vi "SaveTCInfo.vi"() -> ()   [LabVIEW 2019, in "TestSeqClass.lvclass"]
uses:
  testSeq/TestSeqClass.lvclass
  testSeq/TypeDef/TestStepInfo.ctl
  TypeDef/TestInfo.ctl
panel:
  in  "error in (no error) 2":errorcluster
  in  "Save":bool
  in  "AllTestInfoSpec":T1[](array[typedef])
  in  "error in (no error)":errorcluster
  out "error out":errorcluster
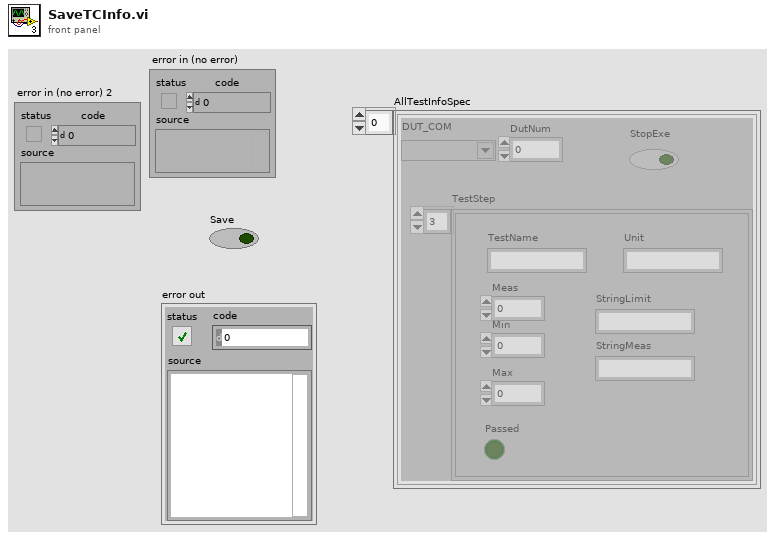
[diagram p1: front panel]
types:
  T1 = typedef "TestInfo.ctl" = cluster{"DUT_COM":refnum<visa-resource-name>, "DutNum":u16, "TestStep":T2[], "StopExe":bool}
  T2 = typedef "TestStepInfo.ctl" = cluster{"TestName":string, "Meas":dbl, "Min ":dbl, "Max":dbl, "Passed":bool, "StringLimit":string, "StringMeas":string, "Unit":string}
  T3 = enum16{"open", "open or create", "create or replace", "create", "open (read only)"}
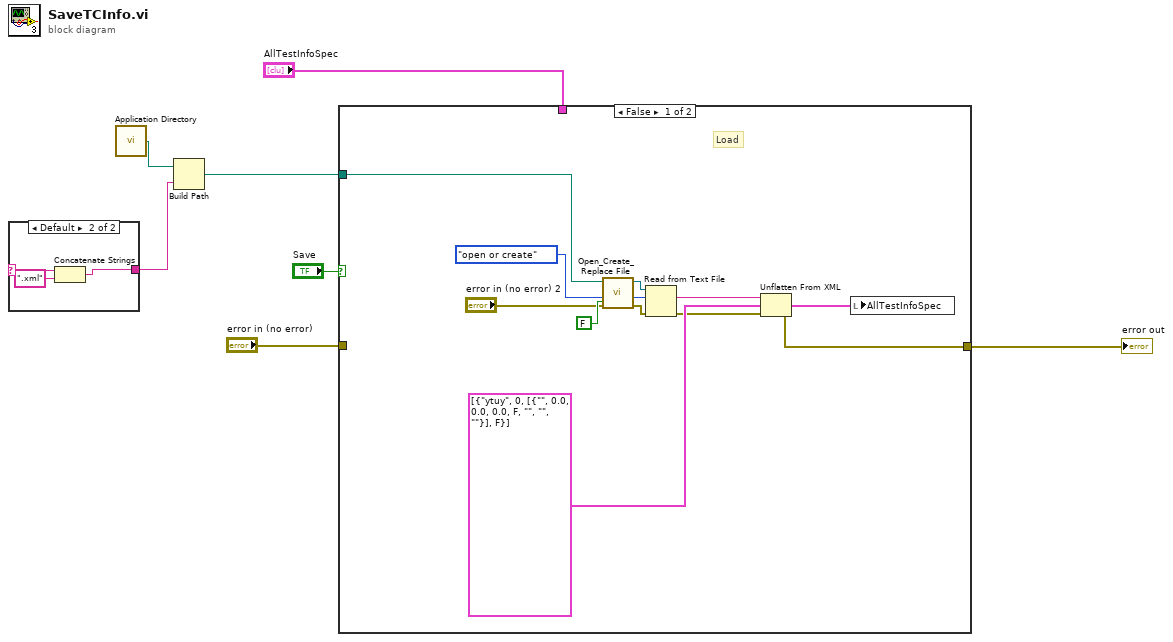
[diagram p0: block diagram]
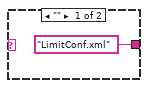
[diagram p2: hidden frame]
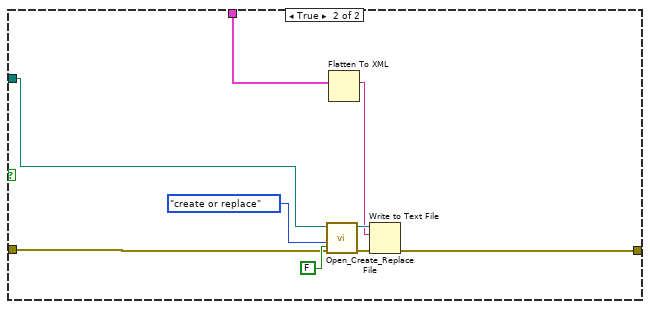
[diagram p3: hidden frame]
diagram:
  n1 = case shown="Default" {
    selector: _ -> [_ w11]
    tunnel: ["LimitConf.xml" ("name or relative path") w9] -> w1
    frame "" {
    }
    frame Default {
      n2 = Concatenate Strings(w11, ".xml" ("string")) -> (w9:string)
    }
  }
  n3 = call <vilib>:"Application Directory.vi"() -> ("Application Directory"=w2:path)
  n4 = Build Path(base path=w2, name or relative path=w1) -> (appended path=w3:path)
  n5 = case shown="False" "Save" {
    tunnel: [w13 w32] -> w7
    tunnel: "error in (no error)" -> [_ w27]
    tunnel: "AllTestInfoSpec" -> [_ w24]
    tunnel: w3 -> [w17 w26]
    frame False {
      # "Load"
      n6 = call <vilib>:"Open_Create_Replace File.vi"("advisory dialog? (display:T)"=FALSE, "error in (no error)"="error in (no error) 2", "function (open:0)"=T3."open or create", "file path"=w17) -> ("error out"=w20:errorcluster, "file size (bytes)"=w18:i32, "refnum"=w19:refnum<file>)  [unwired: 3 in, 2 out]
      n7 = Read from Text File(file (use dialog)=w19, count=w18, error in=w20) -> (text=w16:string, error out=w14:errorcluster)  [unwired: 1 in, 2 out]
      n8 = Unflatten From XML(xml string=w16, type=T1[] [{"DUT_COM"="ytuy", "DutNum"=0, "TestStep"=[{"TestName"="", "Meas"=0.0, "Min "=0.0, "Max"=0.0, "Passed"=FALSE, "StringLimit"="", "StringMeas"="", "Unit"=""}], "StopExe"=FALSE}] ("AllTestInfoSpec"), error in (no error)=w14) -> (value=w12:T1[], error out=w13:errorcluster)
      n9 = local write "AllTestInfoSpec"(w12) -> ()
    }
    frame True {
      n10 = call <vilib>:"Open_Create_Replace File.vi"("advisory dialog? (display:T)"=FALSE, "error in (no error)"=w27, "function (open:0)"=T3."create or replace", "file path"=w26) -> ("error out"=w30:errorcluster, "refnum"=w31:refnum<file>)  [unwired: 3 in, 3 out]
      n11 = Flatten To XML(anything=w24) -> (xml string=w25:string)
      n12 = Write to Text File(file (use dialog)=w31, text=w25, error in=w30) -> (error out=w32:errorcluster)  [unwired: 1 in, 2 out]
    }
  }
  "error out" <- w7
